vi "IRISS_FPGA_IO_v3.1.vi"() -> ()   [LabVIEW 2010]
doc: "This VI contains a basic quadrature decoder which is reset asynchronously upon clicking the reset button."
uses:
  <vilib>/platform/TimedLoop/XDataNode/XDataNode.xnode
  <vilib>/Platform/TimedLoop/XDataNode/nitl_modes.ctl
  <vilib>/Platform/TimedLoop/XDataNode/XDNodeRunTimeDep.lvlib
  <vilib>/Platform/TimedLoop/XDataNode/wakeup.ctl
  <vilib>/Platform/TimedLoop/XDataNode/timing_clust.ctl
  <vilib>/eio/EIONode/EIONode.xnode
  Library/KevinLibraryAll/labview/KevLib01.lvlib
  Library/jmslib.lvlib
panel:
  in  "DIR OCT Mot":bool
  in  "INHB OCT Mot":bool
  out "FAULT OCT Mot":bool
  out "Position OCT Mot":i32
  out "JumpBy2Error OCT Mot":i16
  in  "Reset OCT Mot":bool
  in  "OCT Mot DC":fxp<+,32,0>
  in  "Conn0/DIO15 Button 4":bool
  in  "Conn0/DIO12 Button 1":bool
  in  "Conn0/DIO13 Button 2":bool
  in  "Conn0/DIO14 Button 3":bool
  in  "DIR Y":bool
  in  "INHB Y":bool
  out "FAULT Y":bool
  out "Position Y":i32
  out "JumpBy2Error Y":i16
  in  "Reset Y":bool
  in  "Y DC":fxp<+,32,0>
  in  "DIR X":bool
  in  "INHB X":bool
  out "FAULT X":bool
  out "Position X":i32
  out "JumpBy2Error X":i16
  in  "Reset X":bool
  in  "DIR Z":bool
  in  "INHB Z":bool
  out "FAULT Z":bool
  out "Position Z":i32
  out "JumpBy2Error Z":i16
  in  "Reset Z":bool
  in  "Z DC":fxp<+,32,0>
  in  "X DC":fxp<+,32,0>
  out "samples":i32
  out "Current Monitor":u32[](array[numeric])
  out "Raw Data Response (MSB)":bool[](array[boolean])
  out "Home L4":bool
  out "Home L1":bool
  out "Home L2":bool
  out "Home L3":bool
  in  "Positive Direction C1-4":bool
  out "JumpBy2Error C1-4":i16
  out "32 bit Position C1-4":i32
  in  "Reset C1-4":bool
  in  "Positive Direction C1-1":bool
  out "JumpBy2Error C1-1":i16
  out "32 bit Position C1-1":i32
  in  "Reset C1-1":bool
  out "32 bit Position 17":i32
  in  "Reset 17":bool
  in  "Positive Direction 17":bool
  out "JumpBy2Error 17":i16
  out "32 bit Position 16":i32
  in  "Reset 16":bool
  in  "Positive Direction 16":bool
  out "JumpBy2Error 16":i16
  out "32 bit Position 15":i32
  in  "Reset 15":bool
  in  "Positive Direction 15":bool
  out "JumpBy2Error 15":i16
  out "32 bit Position 14":i32
  in  "Reset 14":bool
  in  "Positive Direction 14":bool
  out "JumpBy2Error 14":i16
  out "32 bit Position 13":i32
  in  "Reset 13":bool
  in  "Positive Direction 13":bool
  out "JumpBy2Error 13":i16
  out "32 bit Position 12":i32
  in  "Reset 12":bool
  in  "Positive Direction 12":bool
  out "JumpBy2Error 12":i16
  out "32 bit Position 11":i32
  in  "Reset 11":bool
  in  "Positive Direction 11":bool
  out "JumpBy2Error 11":i16
  out "32 bit Position 10":i32
  in  "Reset 10":bool
  in  "Positive Direction 10":bool
  out "JumpBy2Error 10":i16
  out "32 bit Position 9":i32
  in  "Reset 9":bool
  in  "Positive Direction 9":bool
  out "JumpBy2Error 9":i16
  out "JumpBy2Error 3":i16
  in  "Positive Direction 3":bool
  out "JumpBy2Error 1":i16
  in  "Positive Direction 1":bool
  out "AI":i16[](array[numeric])
  out "32 bit Position 3":i32
  in  "Reset 3":bool
  in  "AO":i16[](array[numeric])=[0, 0, 0, 0, 0, 0, 0, 0]
  out "32 bit Position 1":i32
  in  "Reset 1":bool
  # "Accurus Buttons"
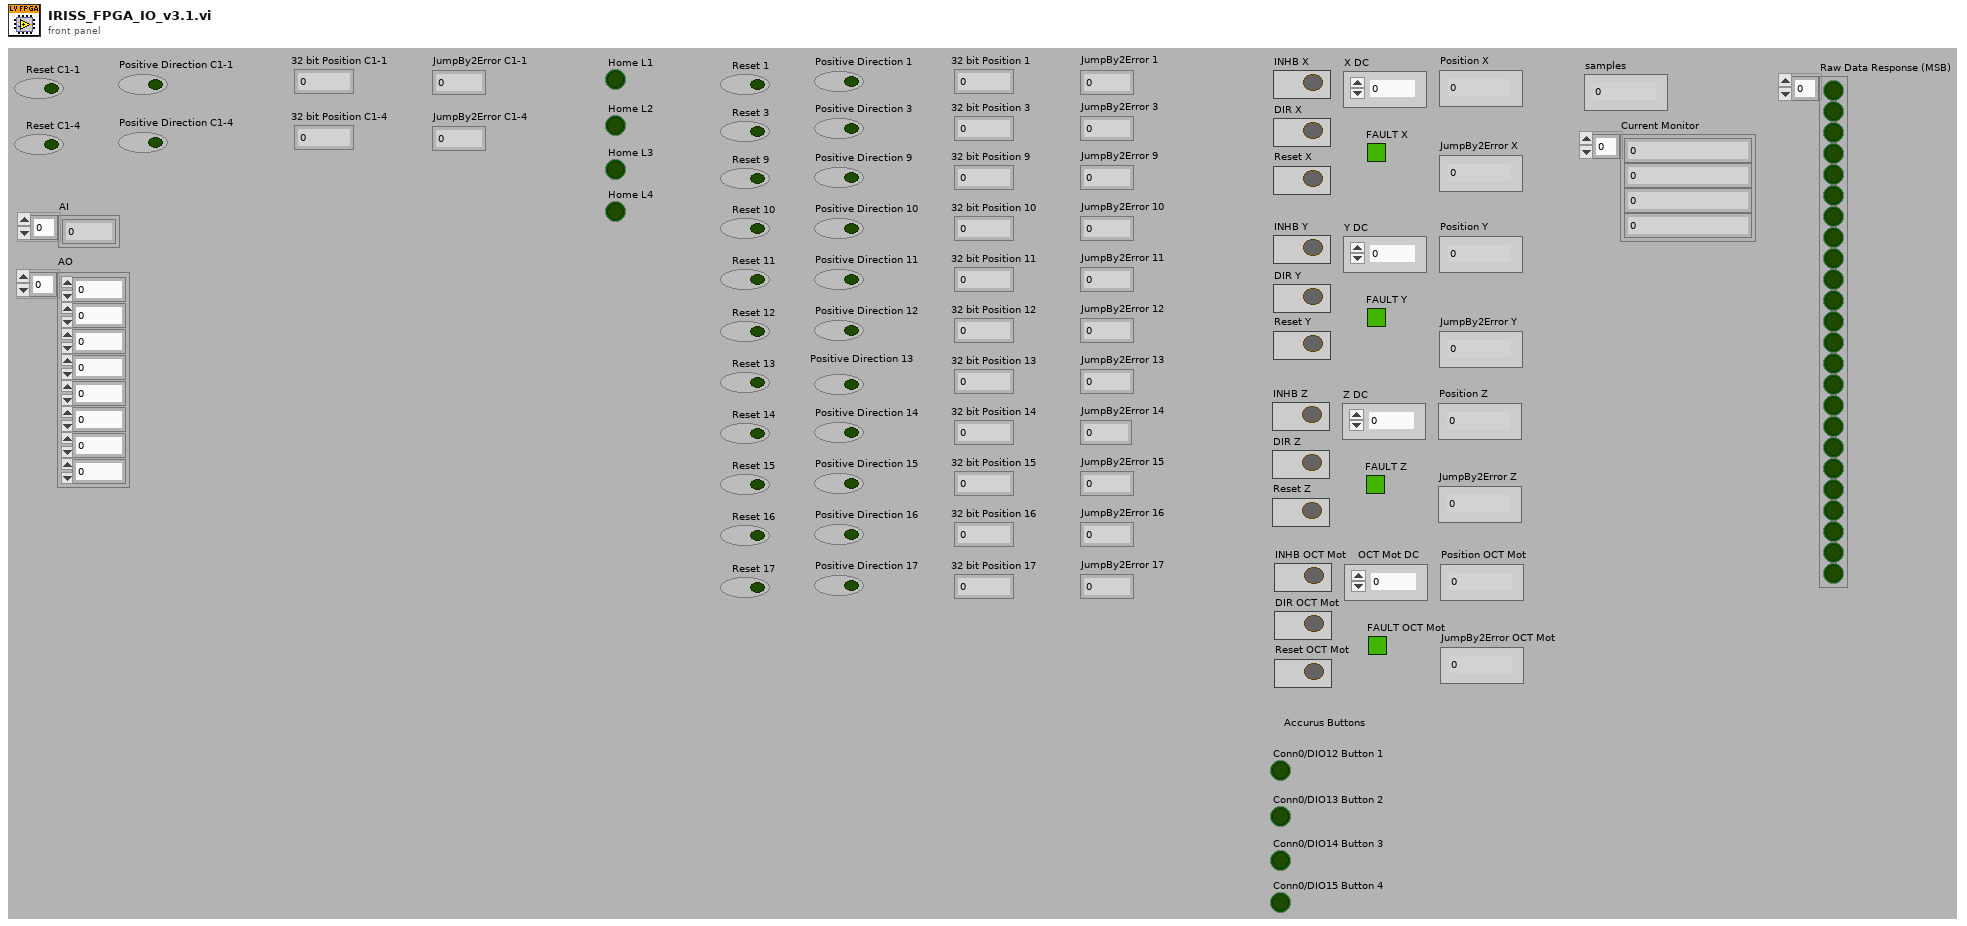
[diagram p1: front panel]
types:
  T1 = typedef "XDNodeRunTimeDep.lvlib/timing_clust.ctl" = cluster{"Expected End [f-1]":u64, "Actual End [f-1]":u64, "Finished Late? [f-1]":bool, "Expected End [i-1]":u64, "Actual End [i-1]":u64, "Finished Late? [i-1]":bool, "Expected Start [i]":u64, "Actual Start [i]":u64, "Expected Start [f]":u64, "Actual Start [f]":u64, "Source Name":string, "Structure Name":string, "Period":i64, "Deadline":i64, "Offset":i64, "Start":i64, "Priority":i32, "Timeout":i32, "Mode":T2, "Wakeup Reason":T3, "Error":errorcluster, "Source Type":string, "Secondary Source Type":string, "Global End Time":u64, "Global Start Time":u64, "Frame Duration":u64, "Iteration Duration":u64, "Assigned CPU":i32, "I/O Scan Engine Mode":u32}
  T2 = typedef "XDNodeRunTimeDep.lvlib/nitl_modes.ctl" = enum32{"No Change", "Process missed periods, maintain original phase", "Discard missed periods, maintain original phase", "Process missed periods, ignore original phase", "Discard missed periods, ignore original phase"}
  T3 = typedef "XDNodeRunTimeDep.lvlib/wakeup.ctl" = enum32{"Normal", "Aborted", "Asynchronous wakeup", "Timing source error", "Timed loop error", "Timeout"}
  T4 = cluster{"PWM In":refnum<k21>, "Direction":refnum<k21>, "Inhibit":refnum<k21>, "Encoder C":refnum<k21>, "Encoder B":refnum<k21>, "Encoder A":refnum<k21>, "Fault":refnum<k21>}
  T5 = cluster{"SCLK":refnum<k21>, "MOSI":refnum<k21>, "MISO":refnum<k21>}
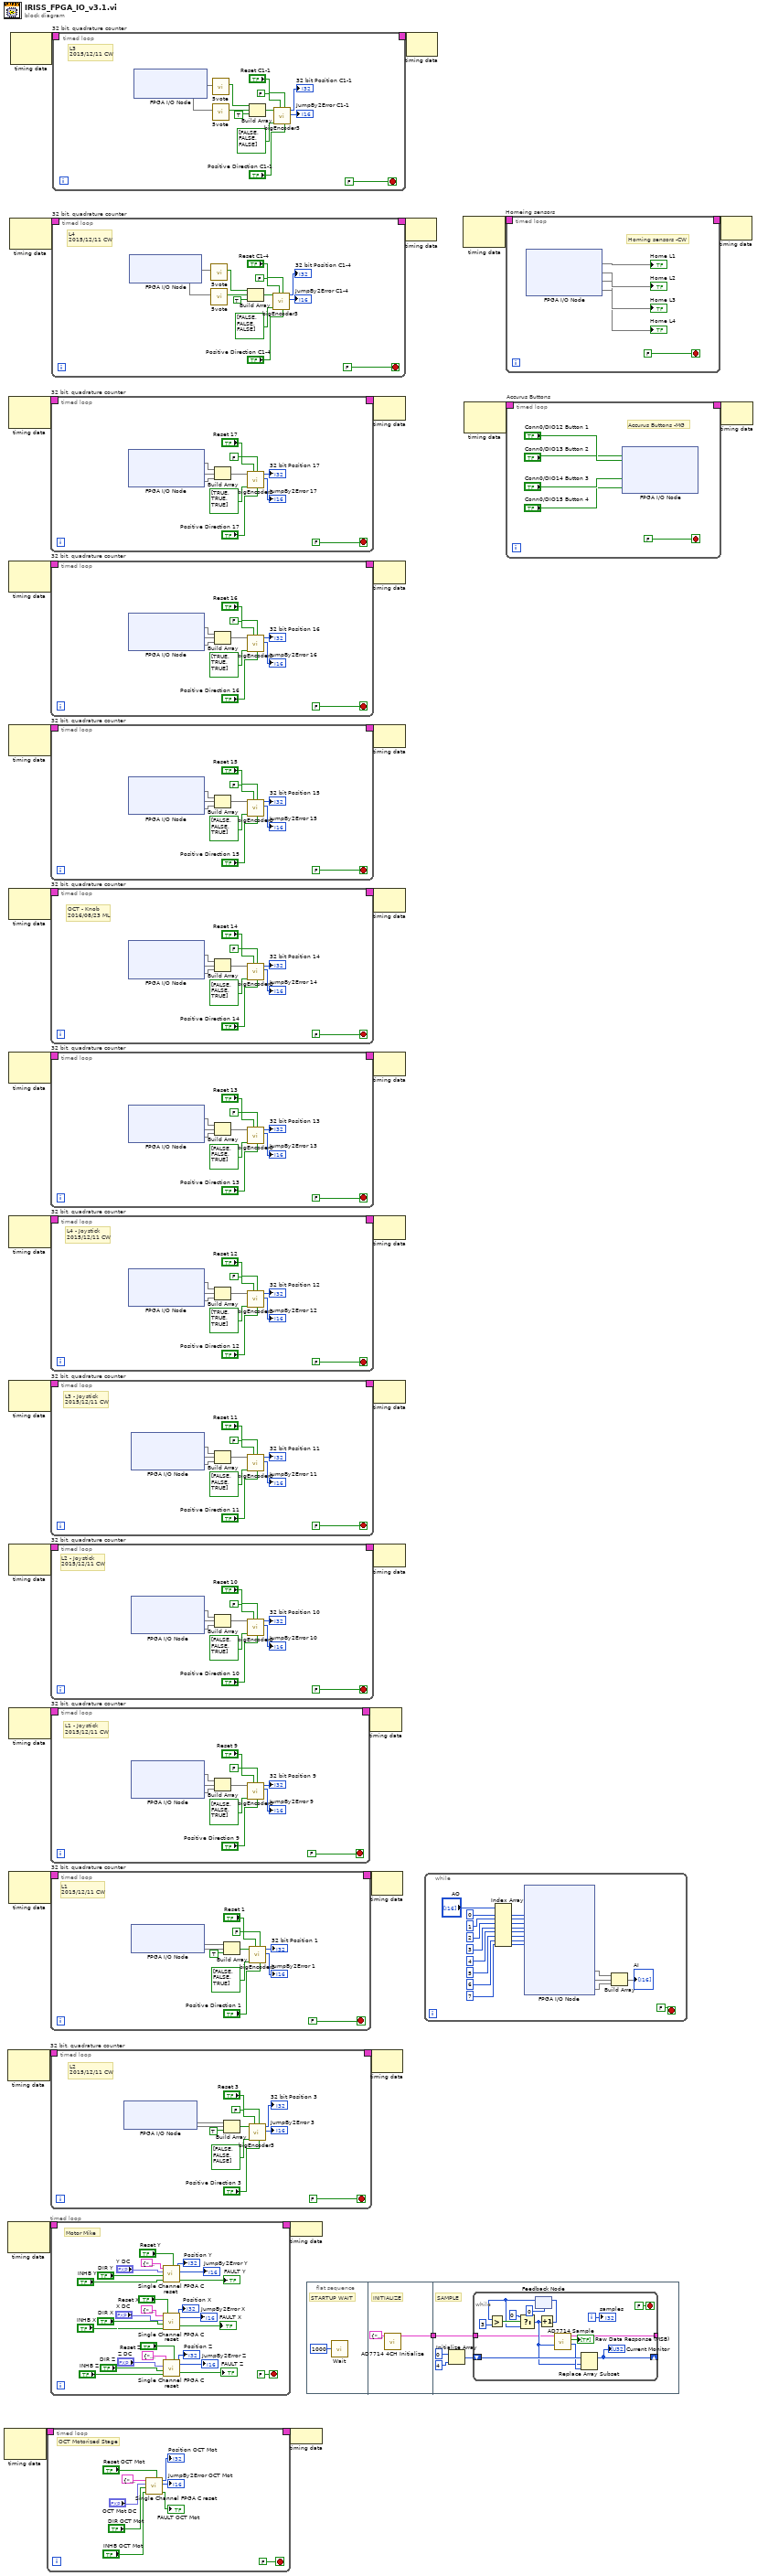
[diagram p0: block diagram]
diagram:
  n1 = node-c288() -> (w2:T1)  [unwired: 2 in]
  n2 = node-c288() -> (w33:T1)  [unwired: 2 out]
  n3 = node-c288() -> (w7:T1)  [unwired: 2 in]
  n4 = node-c288() -> (w15:T1)  [unwired: 2 out]
  n5 = node-c288() -> (w17:T1)  [unwired: 2 out]
  n6 = node-c288() -> (w19:T1)  [unwired: 2 out]
  n7 = node-c288() -> (w21:T1)  [unwired: 2 out]
  n8 = node-c288() -> (w23:T1)  [unwired: 2 out]
  n9 = node-c288() -> (w25:T1)  [unwired: 2 out]
  n10 = node-c288() -> (w27:T1)  [unwired: 2 out]
  n11 = node-c288() -> (w29:T1)  [unwired: 2 out]
  n12 = node-c288() -> (w31:T1)  [unwired: 2 out]
  n13 = node-c288() -> (w34:T1)  [unwired: 2 out]
  n14 = node-c288() -> (w11:T1)  [unwired: 2 out]
  n15 = node-c288() -> (w13:T1)  [unwired: 2 out]
  n16 = timed-loop {
    timing: w2 -> [_]
    timing-out: [_] -> w1
    stop <- FALSE stop-if-true
    # "OCT Motorized Stage"
    n17 = call "Single Channel FPGA C reset.vi"("Reset"="Reset OCT Mot", "INHB"="INHB OCT Mot", "DIR"="DIR OCT Mot", "Duty"="OCT Mot DC", "IO Channels"=T4 {"PWM In"="Connector1/DIO7", "Direction"="Connector1/DIO8", "Inhibit"="Connector1/DIO9", "Encoder C"="Connector1/DIO10", "Encoder B"="Connector1/DIO11", "Encoder A"="Connector1/DIO12", "Fault"="Connector1/DIO13"}) -> ("FAULT"=→"FAULT OCT Mot":bool, "JumpBy2Error"=→"JumpBy2Error OCT Mot":i16, "Position"=→"Position OCT Mot":i32)  [unwired: 4 in]
  }
  n18 = timed-loop "32 bit, quadrature counter" {
    timing-out: [_] -> w32
    timing: w33 -> [_]
    stop <- FALSE stop-if-true
    # "L2\n2015/12/11 CW"
    n19 = xnode "FPGA I/O Node"() -> ("Connector0/DIO2"=w50, "Connector0/DIO3"=w49)  [unwired: 2 in, 2 out]
    n20 = Build Array(w50, w49, TRUE ("element")) -> (w56:bool[])
    n21 = call "bigEncoder3.vi"("Positive Direction"="Positive Direction 3", "ForceReset"="Reset 3", "Allow C Reset?"=FALSE, "Reset Array"=bool[] [FALSE, FALSE, FALSE], "Encoder Array"=w56) -> ("JumpBy2Error"=→"JumpBy2Error 3":i16, "Position"=→"32 bit Position 3":i32)  [unwired: 5 out]
  }
  n22 = timed-loop {
    timing: w7 -> [_]
    timing-out: [_] -> w6
    stop <- FALSE stop-if-true
    # "Motor Mike"
    n23 = call "Single Channel FPGA C reset.vi"("Reset"="Reset Y", "INHB"="INHB Y", "DIR"="DIR Y", "Duty"="Y DC", "IO Channels"=T4 {"PWM In"="Connector1/DIO1", "Direction"="Connector1/DIO2", "Inhibit"="Connector1/DIO3", "Encoder C"="Connector1/DIO4", "Encoder B"="Connector1/DIO5", "Encoder A"="Connector1/DIO6", "Fault"="Connector1/DIO0"}) -> ("FAULT"=→"FAULT Y":bool, "JumpBy2Error"=→"JumpBy2Error Y":i16, "Position"=→"Position Y":i32)  [unwired: 4 in]
    n24 = call "Single Channel FPGA C reset.vi"("Reset"="Reset X", "INHB"="INHB X", "DIR"="DIR X", "Duty"="X DC", "IO Channels"=T4 {"PWM In"="Connector1/DIO20", "Direction"="Connector1/DIO21", "Inhibit"="Connector1/DIO22", "Encoder C"="Connector1/DIO23", "Encoder B"="Connector1/DIO24", "Encoder A"="Connector1/DIO25", "Fault"="Connector1/DIO27"}) -> ("FAULT"=→"FAULT X":bool, "JumpBy2Error"=→"JumpBy2Error X":i16, "Position"=→"Position X":i32)  [unwired: 4 in]
    n25 = call "Single Channel FPGA C reset.vi"("Reset"="Reset Z", "INHB"="INHB Z", "DIR"="DIR Z", "Duty"="Z DC", "IO Channels"=T4 {"PWM In"="Connector1/DIO14", "Direction"="Connector1/DIO15", "Inhibit"="Connector1/DIO16", "Encoder C"="Connector1/DIO17", "Encoder B"="Connector1/DIO18", "Encoder A"="Connector1/DIO19", "Fault"="Connector1/DIO26"}) -> ("FAULT"=→"FAULT Z":bool, "JumpBy2Error"=→"JumpBy2Error Z":i16, "Position"=→"Position Z":i32)  [unwired: 4 in]
  }
  n26 = timed-loop "32 bit, quadrature counter" {
    timing-out: [_] -> w14
    timing: w15 -> [_]
    stop <- FALSE stop-if-true
    n27 = xnode "FPGA I/O Node"() -> ("Connector2/DIO24"=w96, "Connector2/DIO25"=w95, "Connector2/DIO26"=w87)  [unwired: 3 in, 3 out]
    n28 = Build Array(w96, w95, w87) -> (w94:void[])
    n29 = call "bigEncoder3.vi"("Positive Direction"="Positive Direction 17", "ForceReset"="Reset 17", "Allow C Reset?"=FALSE, "Reset Array"=bool[] [TRUE, TRUE, TRUE], "Encoder Array"=w94) -> ("JumpBy2Error"=→"JumpBy2Error 17":i16, "Position"=→"32 bit Position 17":i32)  [unwired: 5 out]
  }
  n30 = timed-loop "32 bit, quadrature counter" {
    timing-out: [_] -> w16
    timing: w17 -> [_]
    stop <- FALSE stop-if-true
    n31 = xnode "FPGA I/O Node"() -> ("Connector2/DIO21"=w109, "Connector2/DIO22"=w108, "Connector2/DIO23"=w100)  [unwired: 3 in, 3 out]
    n32 = Build Array(w109, w108, w100) -> (w107:void[])
    n33 = call "bigEncoder3.vi"("Positive Direction"="Positive Direction 16", "ForceReset"="Reset 16", "Allow C Reset?"=FALSE, "Reset Array"=bool[] [TRUE, TRUE, TRUE], "Encoder Array"=w107) -> ("JumpBy2Error"=→"JumpBy2Error 16":i16, "Position"=→"32 bit Position 16":i32)  [unwired: 5 out]
  }
  n34 = timed-loop "32 bit, quadrature counter" {
    timing-out: [_] -> w18
    timing: w19 -> [_]
    stop <- FALSE stop-if-true
    n35 = xnode "FPGA I/O Node"() -> ("Connector2/DIO18"=w122, "Connector2/DIO19"=w121, "Connector2/DIO20"=w113)  [unwired: 3 in, 3 out]
    n36 = Build Array(w122, w121, w113) -> (w120:void[])
    n37 = call "bigEncoder3.vi"("Positive Direction"="Positive Direction 15", "ForceReset"="Reset 15", "Allow C Reset?"=FALSE, "Reset Array"=bool[] [FALSE, FALSE, TRUE], "Encoder Array"=w120) -> ("JumpBy2Error"=→"JumpBy2Error 15":i16, "Position"=→"32 bit Position 15":i32)  [unwired: 5 out]
  }
  n38 = timed-loop "32 bit, quadrature counter" {
    timing-out: [_] -> w20
    timing: w21 -> [_]
    stop <- FALSE stop-if-true
    # "OCT - Knob\n2016/08/23 ML"
    n39 = xnode "FPGA I/O Node"() -> ("Connector2/DIO15"=w135, "Connector2/DIO16"=w134, "Connector2/DIO17"=w126)  [unwired: 3 in, 3 out]
    n40 = Build Array(w135, w134, w126) -> (w133:void[])
    n41 = call "bigEncoder3.vi"("Positive Direction"="Positive Direction 14", "ForceReset"="Reset 14", "Allow C Reset?"=FALSE, "Reset Array"=bool[] [FALSE, FALSE, TRUE], "Encoder Array"=w133) -> ("JumpBy2Error"=→"JumpBy2Error 14":i16, "Position"=→"32 bit Position 14":i32)  [unwired: 5 out]
  }
  n42 = timed-loop "32 bit, quadrature counter" {
    timing-out: [_] -> w22
    timing: w23 -> [_]
    stop <- FALSE stop-if-true
    n43 = xnode "FPGA I/O Node"() -> ("Connector2/DIO12"=w148, "Connector2/DIO13"=w147, "Connector2/DIO14"=w139)  [unwired: 3 in, 3 out]
    n44 = Build Array(w148, w147, w139) -> (w146:void[])
    n45 = call "bigEncoder3.vi"("Positive Direction"="Positive Direction 13", "ForceReset"="Reset 13", "Allow C Reset?"=FALSE, "Reset Array"=bool[] [FALSE, FALSE, TRUE], "Encoder Array"=w146) -> ("JumpBy2Error"=→"JumpBy2Error 13":i16, "Position"=→"32 bit Position 13":i32)  [unwired: 5 out]
  }
  n46 = timed-loop "32 bit, quadrature counter" {
    timing-out: [_] -> w24
    timing: w25 -> [_]
    stop <- FALSE stop-if-true
    # "L4 - Joystick\n2015/12/11 CW"
    n47 = xnode "FPGA I/O Node"() -> ("Connector2/DIO9"=w161, "Connector2/DIO10"=w160, "Connector2/DIO11"=w152)  [unwired: 3 in, 3 out]
    n48 = Build Array(w161, w160, w152) -> (w159:void[])
    n49 = call "bigEncoder3.vi"("Positive Direction"="Positive Direction 12", "ForceReset"="Reset 12", "Allow C Reset?"=FALSE, "Reset Array"=bool[] [TRUE, TRUE, TRUE], "Encoder Array"=w159) -> ("JumpBy2Error"=→"JumpBy2Error 12":i16, "Position"=→"32 bit Position 12":i32)  [unwired: 5 out]
  }
  n50 = timed-loop "32 bit, quadrature counter" {
    timing-out: [_] -> w26
    timing: w27 -> [_]
    stop <- FALSE stop-if-true
    # "L3 - Joystick\n2015/12/11 CW"
    n51 = xnode "FPGA I/O Node"() -> ("Connector2/DIO6"=w174, "Connector2/DIO7"=w173, "Connector2/DIO8"=w165)  [unwired: 3 in, 3 out]
    n52 = Build Array(w174, w173, w165) -> (w172:void[])
    n53 = call "bigEncoder3.vi"("Positive Direction"="Positive Direction 11", "ForceReset"="Reset 11", "Allow C Reset?"=FALSE, "Reset Array"=bool[] [FALSE, FALSE, TRUE], "Encoder Array"=w172) -> ("JumpBy2Error"=→"JumpBy2Error 11":i16, "Position"=→"32 bit Position 11":i32)  [unwired: 5 out]
  }
  n54 = timed-loop "32 bit, quadrature counter" {
    timing-out: [_] -> w28
    timing: w29 -> [_]
    stop <- FALSE stop-if-true
    # "L2 - Joystick\n2015/12/11 CW"
    n55 = xnode "FPGA I/O Node"() -> ("Connector2/DIO3"=w187, "Connector2/DIO4"=w186, "Connector2/DIO5"=w178)  [unwired: 3 in, 3 out]
    n56 = Build Array(w187, w186, w178) -> (w185:void[])
    n57 = call "bigEncoder3.vi"("Positive Direction"="Positive Direction 10", "ForceReset"="Reset 10", "Allow C Reset?"=FALSE, "Reset Array"=bool[] [FALSE, FALSE, TRUE], "Encoder Array"=w185) -> ("JumpBy2Error"=→"JumpBy2Error 10":i16, "Position"=→"32 bit Position 10":i32)  [unwired: 5 out]
  }
  n58 = timed-loop "32 bit, quadrature counter" {
    timing-out: [_] -> w30
    timing: w31 -> [_]
    stop <- FALSE stop-if-true
    # "L1 - Joystick\n2015/12/11 CW"
    n59 = xnode "FPGA I/O Node"() -> ("Connector2/DIO0"=w200, "Connector2/DIO1"=w199, "Connector2/DIO2"=w191)  [unwired: 3 in, 3 out]
    n60 = Build Array(w200, w199, w191) -> (w198:void[])
    n61 = call "bigEncoder3.vi"("Positive Direction"="Positive Direction 9", "ForceReset"="Reset 9", "Allow C Reset?"=FALSE, "Reset Array"=bool[] [FALSE, FALSE, TRUE], "Encoder Array"=w198) -> ("JumpBy2Error"=→"JumpBy2Error 9":i16, "Position"=→"32 bit Position 9":i32)  [unwired: 5 out]
  }
  n62 = timed-loop "32 bit, quadrature counter" {
    timing-out: [_] -> w35
    timing: w34 -> [_]
    stop <- FALSE stop-if-true
    # "L1\n2015/12/11 CW"
    n63 = xnode "FPGA I/O Node"() -> ("Connector0/DIO0"=w213, "Connector0/DIO1"=w212)  [unwired: 2 in, 2 out]
    n64 = Build Array(w213, w212, TRUE ("element")) -> (w211:bool[])
    n65 = call "bigEncoder3.vi"("Positive Direction"="Positive Direction 1", "ForceReset"="Reset 1", "Allow C Reset?"=FALSE, "Reset Array"=bool[] [FALSE, FALSE, TRUE], "Encoder Array"=w211) -> ("JumpBy2Error"=→"JumpBy2Error 1":i16, "Position"=→"32 bit Position 1":i32)  [unwired: 5 out]
  }
  n66 = timed-loop "32 bit, quadrature counter" {
    timing-out: [_] -> w10
    timing: w11 -> [_]
    stop <- FALSE stop-if-true
    # "L4\n2015/12/11 CW"
    n67 = xnode "FPGA I/O Node"() -> ("Connector0/DIO6"=w220, "Connector0/DIO7"=w219)  [unwired: 2 in, 2 out]
    n68 = call "5vote.vi"("Input"=w220) -> ("vote5"=w217:bool)  [unwired: 10 in]
    n69 = call "5vote.vi"("Input"=w219) -> ("vote5"=w218:bool)  [unwired: 10 in]
    n70 = Build Array(w217, w218, TRUE ("element")) -> (w228:bool[])
    n71 = call "bigEncoder3.vi"("Positive Direction"="Positive Direction C1-4", "ForceReset"="Reset C1-4", "Allow C Reset?"=FALSE, "Reset Array"=bool[] [FALSE, FALSE, FALSE], "Encoder Array"=w228) -> ("JumpBy2Error"=→"JumpBy2Error C1-4":i16, "Position"=→"32 bit Position C1-4":i32)  [unwired: 5 out]
  }
  n72 = timed-loop "32 bit, quadrature counter" {
    timing-out: [_] -> w12
    timing: w13 -> [_]
    stop <- FALSE stop-if-true
    # "L3\n2015/12/11 CW"
    n73 = xnode "FPGA I/O Node"() -> ("Connector0/DIO4"=w235, "Connector0/DIO5"=w234)  [unwired: 2 in, 2 out]
    n74 = call "5vote.vi"("Input"=w235) -> ("vote5"=w232:bool)  [unwired: 10 in]
    n75 = call "5vote.vi"("Input"=w234) -> ("vote5"=w233:bool)  [unwired: 10 in]
    n76 = Build Array(w232, w233, TRUE ("element")) -> (w243:bool[])
    n77 = call "bigEncoder3.vi"("Positive Direction"="Positive Direction C1-1", "ForceReset"="Reset C1-1", "Allow C Reset?"=FALSE, "Reset Array"=bool[] [FALSE, FALSE, FALSE], "Encoder Array"=w243) -> ("JumpBy2Error"=→"JumpBy2Error C1-1":i16, "Position"=→"32 bit Position C1-1":i32)  [unwired: 5 out]
  }
  n78 = node-c288(w6) -> ()
  n79 = node-c288(w1) -> ()
  n80 = flat-sequence {
    tunnel: [w248] -> w5
    tunnel: w5 -> [w250]
    frame #0 {
      # "STARTUP WAIT"
      n81 = call "Wait"("Count(uSec)"=u32 1000) -> ()  [unwired: 1 out]
    }
    frame #1 {
      # "INITIALIZE"
      n82 = call "AD7714 4CH Initialize.vi"("I/O Cluster In"=T5 {"SCLK"="Connector1/DIO29", "MOSI"="Connector1/DIO35", "MISO"="Connector1/DIO31"}) -> ("I/O Cluster Out"=w248:T5)  [unwired: 10 in]
    }
    frame #2 {
      # "SAMPLE"
      n83 = Initialize Array(u32 0, 4 ("dimension size")) -> (w251:u32[])
      n84 = while {
        shift-right: [w259] -> _
        shift-left: w251 -> [w260]
        tunnel: w250 -> [w256]
        tunnel: [w255] -> _
        i -> [w267]
        stop <- FALSE stop-if-true
        n85 = feedback #1(i16 0) -> (w263:i16)
        n86 = Greater?(x=w263, y=i16 3) -> (0:w264:bool)
        n87 = Select(t=i16 0, s=w264, f=w263) -> (s? t:f=w257:i16)
        n88 = Increment(x=w257) -> (x+1=w261:i16)
        n89 = feedback-in #1(w261) -> ()
        n90 = call "AD7714 Sample.vi"("Channel"=w257, "I/O Cluster In"=w256) -> ("Data"=w258:u32, "Raw Data Response (MSB)"=→"Raw Data Response (MSB)":bool[], "I/O Cluster Out"=w255:T5)  [unwired: 7 in]
        n91 = Replace Array Subset(array=w260, new element=w258, index=w257) -> (w259:u32[])
        "Current Monitor" <- w259
        "samples" <- w267
      }
    }
  }
  n92 = node-c288(w30) -> ()  [unwired: 1 out]
  n93 = node-c288(w35) -> ()  [unwired: 1 out]
  n94 = node-c288(w32) -> ()  [unwired: 1 out]
  n95 = node-c288(w14) -> ()  [unwired: 1 out]
  n96 = node-c288(w16) -> ()  [unwired: 1 out]
  n97 = node-c288(w18) -> ()  [unwired: 1 out]
  n98 = node-c288(w20) -> ()  [unwired: 1 out]
  n99 = node-c288(w22) -> ()  [unwired: 1 out]
  n100 = node-c288(w24) -> ()  [unwired: 1 out]
  n101 = node-c288(w26) -> ()  [unwired: 1 out]
  n102 = node-c288(w28) -> ()  [unwired: 1 out]
  n103 = node-c288(w10) -> ()  [unwired: 1 out]
  n104 = node-c288(w12) -> ()  [unwired: 1 out]
  n105 = while {
    stop <- FALSE stop-if-true
    n106 = Index Array(array="AO", index #1=0 ("index"), index #2=1 ("index"), index #3=2 ("index"), index #4=3 ("index"), index #5=4 ("index"), index #6=5 ("index"), index #7=6 ("index"), index #8=7 ("index")) -> (element #1=w281:i16, element #2=w280:i16, element #3=w279:i16, element #4=w278:i16, element #5=w277:i16, element #6=w276:i16, element #7=w275:i16, element #8=w274:i16)
    n107 = xnode "FPGA I/O Node"("Connector0/AO0"=w281, "Connector0/AO1"=w280, "Connector0/AO2"=w279, "Connector0/AO3"=w278, "Connector0/AO4"=w277, "Connector0/AO5"=w276, "Connector0/AO6"=w275, "Connector0/AO7"=w274) -> ("Connector0/AI0"=w272, "Connector0/AI1"=w271, "Connector0/AI2"=w269)  [unwired: 11 in, 11 out]
    n108 = Build Array(w272, w271, w269) -> (→"AI":void[])
  }
  n109 = node-c288() -> (w9:T1)  [unwired: 2 out]
  n110 = node-c288() -> (w4:T1)  [unwired: 2 out]
  n111 = timed-loop "Homeing sensors" {
    timing-out: [_] -> w8
    timing: w9 -> [_]
    stop <- FALSE stop-if-true
    # "Homing sensors -CW"
    n112 = xnode "FPGA I/O Node"() -> ("Connector0/DIO8"=→"Home L1", "Connector0/DIO9"=→"Home L2", "Connector0/DIO10"=→"Home L3", "Connector0/DIO11"=→"Home L4")  [unwired: 4 in, 4 out]
  }
  n113 = timed-loop "Accurus Buttons" {
    timing-out: [_] -> w3
    timing: w4 -> [_]
    stop <- FALSE stop-if-true
    # "Accurus Buttons -MG"
    n114 = xnode "FPGA I/O Node"("Connector0/DIO12"="Conn0/DIO12 Button 1", "Connector0/DIO13"="Conn0/DIO13 Button 2", "Connector0/DIO14"="Conn0/DIO14 Button 3", "Connector0/DIO15"="Conn0/DIO15 Button 4") -> ()  [unwired: 4 in, 4 out]
  }
  n115 = node-c288(w8) -> ()  [unwired: 1 out]
  n116 = node-c288(w3) -> ()  [unwired: 1 out]
